vi "Read Logs.vi"() -> ()   [LabVIEW 2020]
panel:
  out "Current Godograph store":cluster{"Y":dbl[], "Y":dbl[]}[](array[cluster])
  out "Voltage Godograph store":cluster{"Y":dbl[], "Y":dbl[]}[](array[cluster])
  out "Current Park Spectrum store":waveform(dbl)[](array[waveform])
  out "Voltage Park Spectrum store":waveform(dbl)[](array[waveform])
  out "Current Spectrum store":waveform(dbl)[](array[waveform])
  out "Voltage Spectrum store":waveform(dbl)[](array[waveform])
  out "Voltage store":waveform(dbl)[](array[waveform])
  out "Current store":waveform(dbl)[](array[waveform])
  in  "Hold":bool
  in  "Plot Selector":u16(ring) items=["Current", "Voltage", "Current Godograph", "Voltage Godograph", "Current Spectrum", "Voltage Spectrum", "Current Park Spectrum", "Voltage Park Spectrum"]
  in  "Choose file":bool
  out "Current Godograph":cluster{"Y":dbl[], "Y":dbl[]}[](graph)
  out "Voltage Godograph":cluster{"Y":dbl[], "Y":dbl[]}[](graph)
  out "Voltage Park Spectrum":waveform(dbl)[](graph)
  out "Current Park Spectrum":waveform(dbl)[](graph)
  out "Current Spectrum":waveform(dbl)[](graph)
  out "Voltage Spectrum":waveform(dbl)[](graph)
  out "Current":waveform(dbl)[](graph)
  out "Voltage":waveform(dbl)[](graph)
  out "error out":errorcluster
types:
  T1 = enum16{"Always On", "Always Off", "Off While Running"}
  T2 = typedef "LVPositionTypeDef.ctl" = cluster{"Left":i32, "Top":i32}
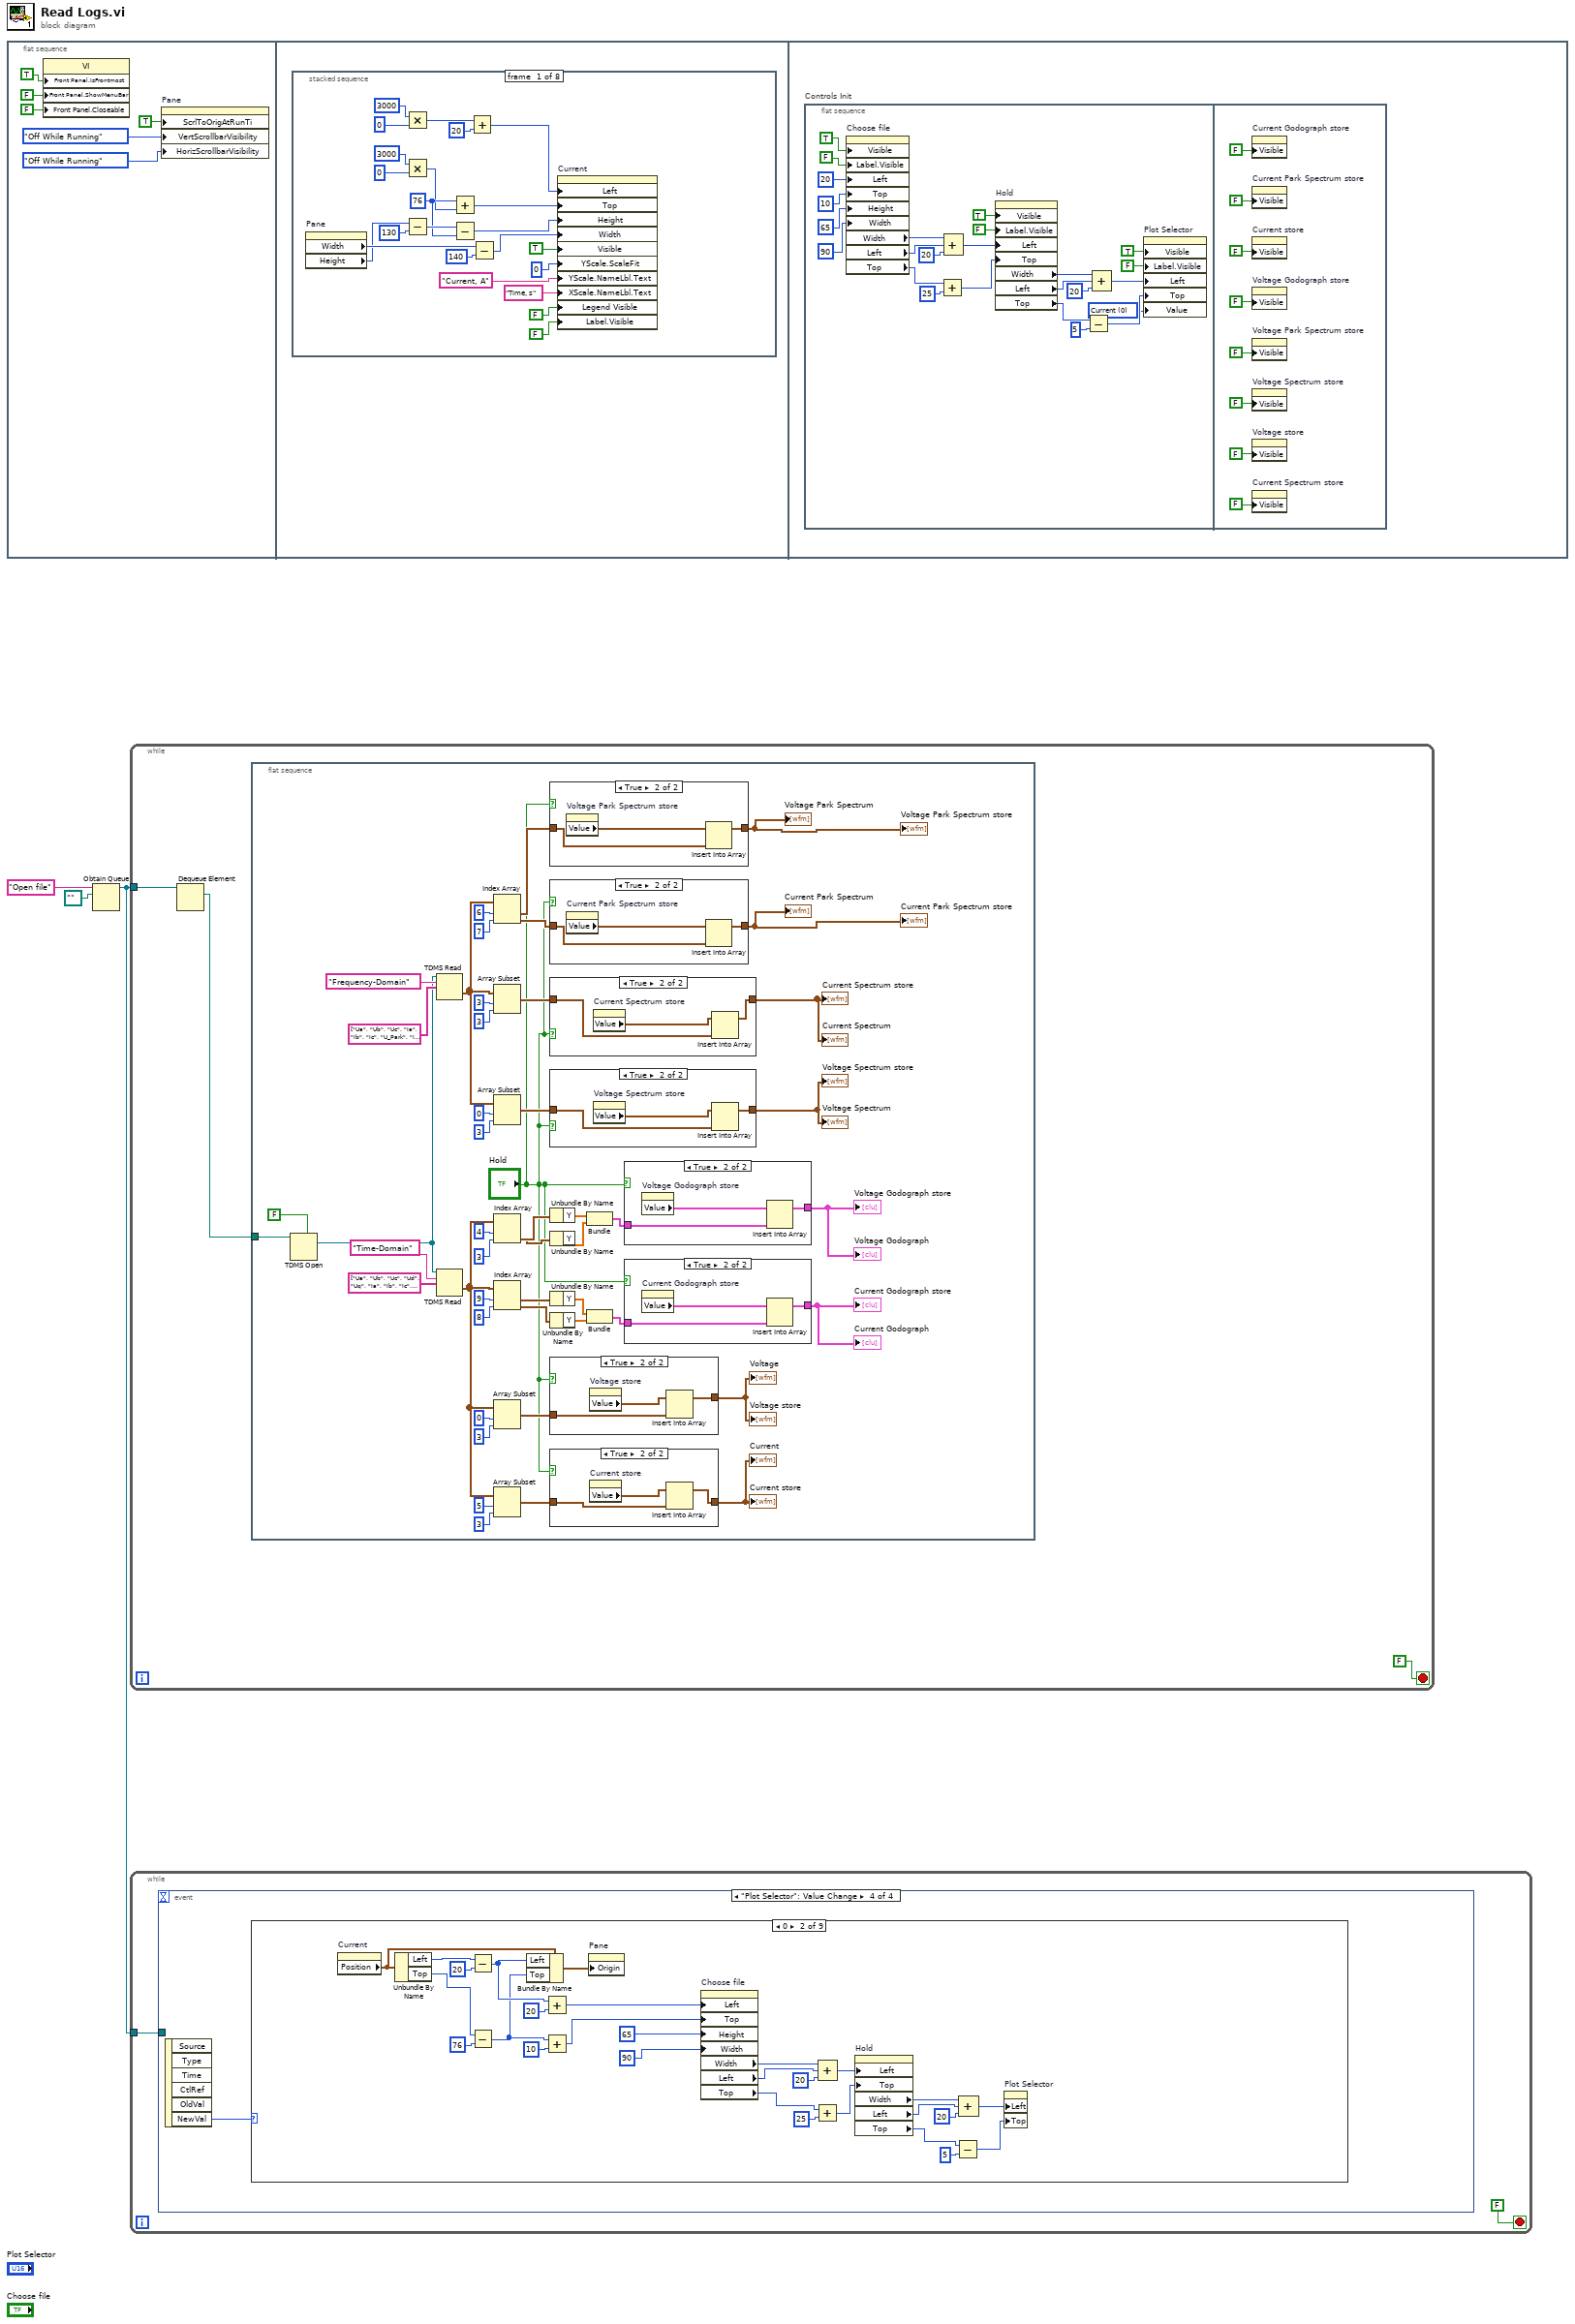
[diagram p0: block diagram]
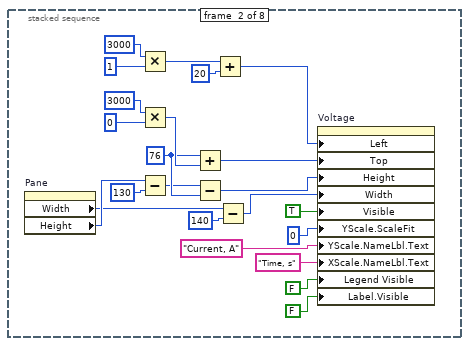
[diagram p2: hidden frame]
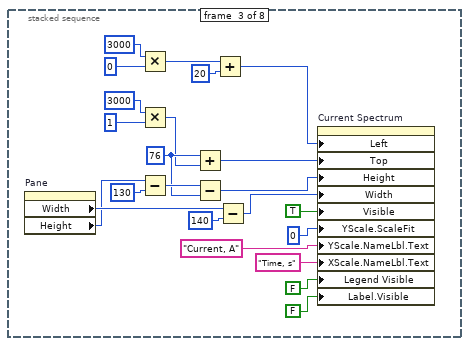
[diagram p3: hidden frame]
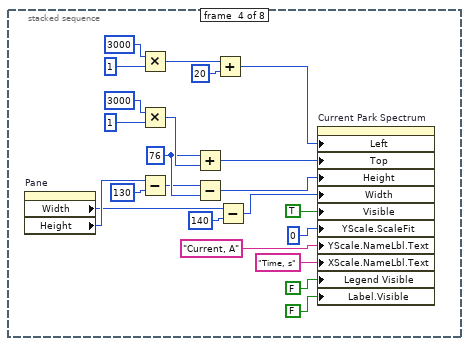
[diagram p4: hidden frame]
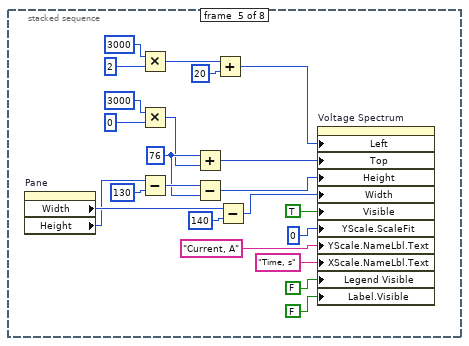
[diagram p5: hidden frame]
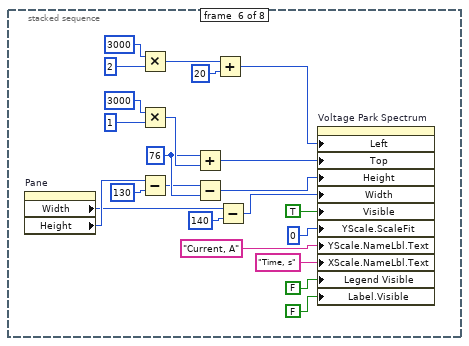
[diagram p6: hidden frame]
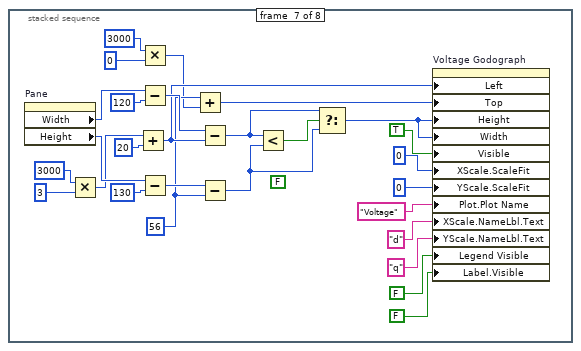
[diagram p7: hidden frame]
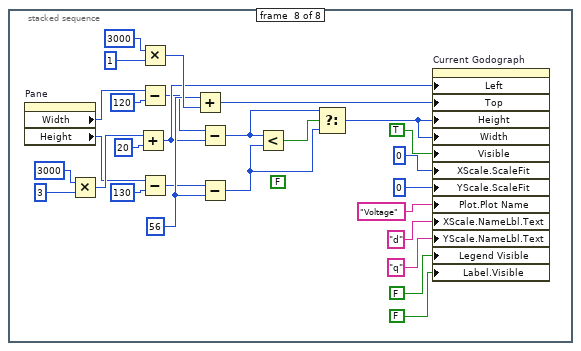
[diagram p8: hidden frame]
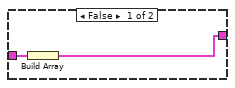
[diagram p9: hidden frame]
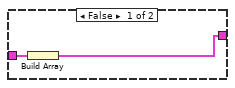
[diagram p10: hidden frame]
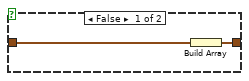
[diagram p11: hidden frame]
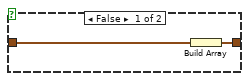
[diagram p12: hidden frame]
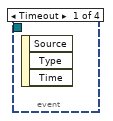
[diagram p17: hidden frame]
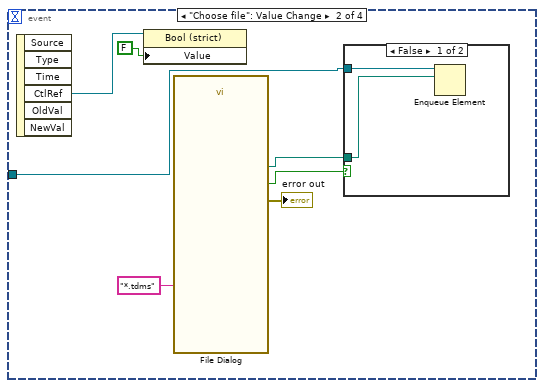
[diagram p18: hidden frame]
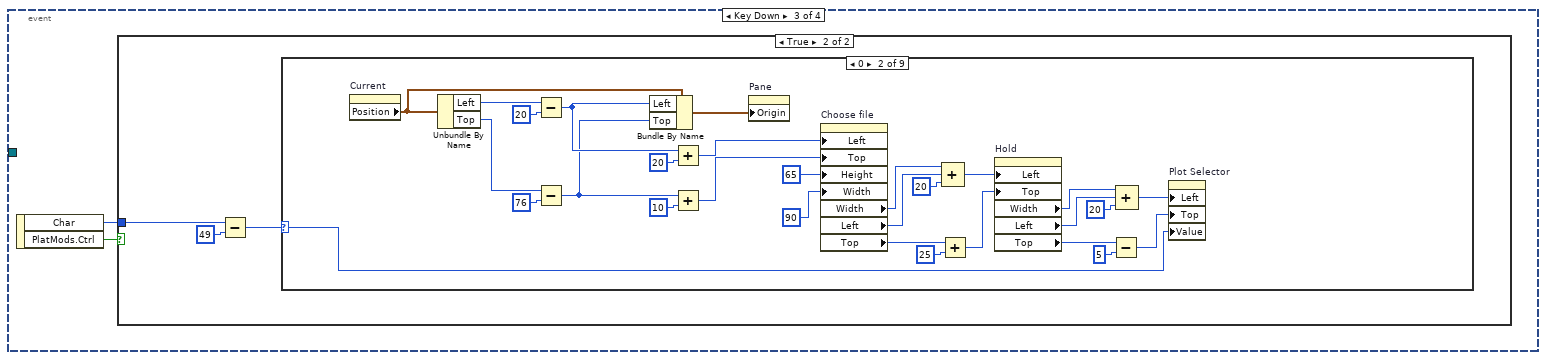
[diagram p20: hidden frame]
diagram:
  n1 = flat-sequence {
    frame #0 {
      n2 = property class="VI"("Front Panel.IsFrontmost"=TRUE ("Front Panel Window:Is Frontmost"), "Front Panel.ShowMenuBar"=FALSE ("Front Panel Window:Show Menu Bar"), "Front Panel.Closeable"=FALSE ("Front Panel Window:Closeable")) -> ()  [unwired: 2 in, 2 out]
      n3 = property on="Pane" class="Pane"("ScrlToOrigAtRunTi"=TRUE ("Scroll To Origin At Run Time"), "VertScrollbarVisibility"=T1."Off While Running" ("Vertical Scrollbar Visibility"), "HorizScrollbarVisibility"=T1."Off While Running" ("Horizontal Scrollbar Visibility")) -> ()  [unwired: 2 in, 2 out]
    }
    frame #1 {
      n4 = stacked-sequence {
        frame #0 {
          w13 = 76 ("Position:Top")
          n5 = property on="Pane" class="Pane"() -> ("Width"=w31:u32, "Height"=w25:u32)  [unwired: 2 in, 2 out]
          n6 = Multiply(x=3000, y=0 ("Position:Left")) -> (x*y=w19:i32)
          n7 = Multiply(x=3000, y=0 ("Position:Left")) -> (x*y=w12:i32)
          n8 = Subtract(x=w25, y=u32 130) -> (x-y=w29:u32)
          n9 = Add(x=w13, y=w12) -> (x+y=w14:i32)
          n10 = Subtract(x=w29, y=w13) -> (x-y=w27:u32)
          n11 = Add(x=w19, y=20 ("Position:Left")) -> (x+y=w21:i32)
          n12 = Subtract(x=w31, y=u32 140) -> (x-y=w11:u32)
          n13 = property on="Current" class="WFGraph (strict)"("Left"=w21, "Top"=w14, "Height"=w27, "Width"=w11, "Visible"=TRUE, "YScale.ScaleFit"=u8 0 ("Y Scale.Scale Fit"), "YScale.NameLbl.Text"="Current, A" ("Y Scale.Name Label.Text"), "XScale.NameLbl.Text"="Time, s" ("X Scale.Name Label.Text"), "Legend Visible"=FALSE ("Legend:Visible"), "Label.Visible"=FALSE) -> ()  [unwired: 2 in, 2 out]
        }
        frame #1 {
          w54 = 76 ("Position:Top")
          n14 = property on="Pane" class="Pane"() -> ("Width"=w36:u32, "Height"=w42:u32)  [unwired: 2 in, 2 out]
          n15 = Multiply(x=3000, y=1 ("Position:Left")) -> (x*y=w48:i32)
          n16 = Multiply(x=3000, y=0 ("Position:Left")) -> (x*y=w55:i32)
          n17 = Subtract(x=w42, y=u32 130) -> (x-y=w38:u32)
          n18 = Add(x=w54, y=w55) -> (x+y=w53:i32)
          n19 = Subtract(x=w38, y=w54) -> (x-y=w40:u32)
          n20 = Add(x=w48, y=20 ("Position:Left")) -> (x+y=w46:i32)
          n21 = Subtract(x=w36, y=u32 140) -> (x-y=w34:u32)
          n22 = property on="Voltage" class="WFGraph (strict)"("Left"=w46, "Top"=w53, "Height"=w40, "Width"=w34, "Visible"=TRUE, "YScale.ScaleFit"=u8 0 ("Y Scale.Scale Fit"), "YScale.NameLbl.Text"="Current, A" ("Y Scale.Name Label.Text"), "XScale.NameLbl.Text"="Time, s" ("X Scale.Name Label.Text"), "Legend Visible"=FALSE ("Legend:Visible"), "Label.Visible"=FALSE) -> ()  [unwired: 2 in, 2 out]
        }
        frame #2 {
          w60 = 76 ("Position:Top")
          n23 = property on="Pane" class="Pane"() -> ("Width"=w77:u32, "Height"=w71:u32)  [unwired: 2 in, 2 out]
          n24 = Multiply(x=3000, y=0 ("Position:Left")) -> (x*y=w65:i32)
          n25 = Multiply(x=3000, y=1 ("Position:Left")) -> (x*y=w59:i32)
          n26 = Subtract(x=w71, y=u32 130) -> (x-y=w75:u32)
          n27 = Add(x=w60, y=w59) -> (x+y=w61:i32)
          n28 = Subtract(x=w75, y=w60) -> (x-y=w73:u32)
          n29 = Add(x=w65, y=20 ("Position:Left")) -> (x+y=w67:i32)
          n30 = Subtract(x=w77, y=u32 140) -> (x-y=w57:u32)
          n31 = property on="Current Spectrum" class="WFGraph (strict)"("Left"=w67, "Top"=w61, "Height"=w73, "Width"=w57, "Visible"=TRUE, "YScale.ScaleFit"=u8 0 ("Y Scale.Scale Fit"), "YScale.NameLbl.Text"="Current, A" ("Y Scale.Name Label.Text"), "XScale.NameLbl.Text"="Time, s" ("X Scale.Name Label.Text"), "Legend Visible"=FALSE ("Legend:Visible"), "Label.Visible"=FALSE) -> ()  [unwired: 2 in, 2 out]
        }
        frame #3 {
          w99 = 76 ("Position:Top")
          n32 = property on="Pane" class="Pane"() -> ("Width"=w82:u32, "Height"=w88:u32)  [unwired: 2 in, 2 out]
          n33 = Multiply(x=3000, y=1 ("Position:Left")) -> (x*y=w94:i32)
          n34 = Multiply(x=3000, y=1 ("Position:Left")) -> (x*y=w100:i32)
          n35 = Subtract(x=w88, y=u32 130) -> (x-y=w84:u32)
          n36 = Add(x=w99, y=w100) -> (x+y=w98:i32)
          n37 = Subtract(x=w84, y=w99) -> (x-y=w86:u32)
          n38 = Add(x=w94, y=20 ("Position:Left")) -> (x+y=w92:i32)
          n39 = Subtract(x=w82, y=u32 140) -> (x-y=w80:u32)
          n40 = property on="Current Park Spectrum" class="WFGraph (strict)"("Left"=w92, "Top"=w98, "Height"=w86, "Width"=w80, "Visible"=TRUE, "YScale.ScaleFit"=u8 0 ("Y Scale.Scale Fit"), "YScale.NameLbl.Text"="Current, A" ("Y Scale.Name Label.Text"), "XScale.NameLbl.Text"="Time, s" ("X Scale.Name Label.Text"), "Legend Visible"=FALSE ("Legend:Visible"), "Label.Visible"=FALSE) -> ()  [unwired: 2 in, 2 out]
        }
        frame #4 {
          w106 = 76 ("Position:Top")
          n41 = property on="Pane" class="Pane"() -> ("Width"=w123:u32, "Height"=w117:u32)  [unwired: 2 in, 2 out]
          n42 = Multiply(x=3000, y=2 ("Position:Left")) -> (x*y=w111:i32)
          n43 = Multiply(x=3000, y=0 ("Position:Left")) -> (x*y=w105:i32)
          n44 = Subtract(x=w117, y=u32 130) -> (x-y=w121:u32)
          n45 = Add(x=w106, y=w105) -> (x+y=w107:i32)
          n46 = Subtract(x=w121, y=w106) -> (x-y=w119:u32)
          n47 = Add(x=w111, y=20 ("Position:Left")) -> (x+y=w113:i32)
          n48 = Subtract(x=w123, y=u32 140) -> (x-y=w103:u32)
          n49 = property on="Voltage Spectrum" class="WFGraph (strict)"("Left"=w113, "Top"=w107, "Height"=w119, "Width"=w103, "Visible"=TRUE, "YScale.ScaleFit"=u8 0 ("Y Scale.Scale Fit"), "YScale.NameLbl.Text"="Current, A" ("Y Scale.Name Label.Text"), "XScale.NameLbl.Text"="Time, s" ("X Scale.Name Label.Text"), "Legend Visible"=FALSE ("Legend:Visible"), "Label.Visible"=FALSE) -> ()  [unwired: 2 in, 2 out]
        }
        frame #5 {
          w145 = 76 ("Position:Top")
          n50 = property on="Pane" class="Pane"() -> ("Width"=w128:u32, "Height"=w134:u32)  [unwired: 2 in, 2 out]
          n51 = Multiply(x=3000, y=2 ("Position:Left")) -> (x*y=w140:i32)
          n52 = Multiply(x=3000, y=1 ("Position:Left")) -> (x*y=w146:i32)
          n53 = Subtract(x=w134, y=u32 130) -> (x-y=w130:u32)
          n54 = Add(x=w145, y=w146) -> (x+y=w144:i32)
          n55 = Subtract(x=w130, y=w145) -> (x-y=w132:u32)
          n56 = Add(x=w140, y=20 ("Position:Left")) -> (x+y=w138:i32)
          n57 = Subtract(x=w128, y=u32 140) -> (x-y=w126:u32)
          n58 = property on="Voltage Park Spectrum" class="WFGraph (strict)"("Left"=w138, "Top"=w144, "Height"=w132, "Width"=w126, "Visible"=TRUE, "YScale.ScaleFit"=u8 0 ("Y Scale.Scale Fit"), "YScale.NameLbl.Text"="Current, A" ("Y Scale.Name Label.Text"), "XScale.NameLbl.Text"="Time, s" ("X Scale.Name Label.Text"), "Legend Visible"=FALSE ("Legend:Visible"), "Label.Visible"=FALSE) -> ()  [unwired: 2 in, 2 out]
        }
        frame #6 {
          (unwired) FALSE ("Visible")
          w150 = 56 ("Position:Top")
          n59 = property on="Pane" class="Pane"() -> ("Width"=w169:u32, "Height"=w166:u32)  [unwired: 2 in, 2 out]
          n60 = Multiply(x=3000, y=3 ("Position:Left")) -> (x*y=w153:i32)
          n61 = Add(x=w153, y=20 ("value")) -> (x+y=w161:i32)
          n62 = Multiply(x=3000, y=0 ("Position:Left")) -> (x*y=w149:i32)
          n63 = Subtract(x=w169, y=u32 120) -> (x-y=w173:u32)
          n64 = Subtract(x=w166, y=u32 130) -> (x-y=w172:u32)
          n65 = Add(x=w150, y=w149) -> (x+y=w148:i32)
          n66 = Subtract(x=w173, y=w161) -> (x-y=w167:u32)
          n67 = Subtract(x=w172, y=w150) -> (x-y=w165:u32)
          n68 = Less?(x=w167, y=w165) -> (x < y?=w170:bool)
          n69 = Select(t=w167, s=w170, f=w165) -> (s? t:f=w168:u32)
          n70 = property on="Voltage Godograph" class="XYGraph (strict)"("Left"=w161, "Top"=w148, "Height"=w168, "Width"=w168, "Visible"=TRUE, "XScale.ScaleFit"=u8 0 ("X Scale.Scale Fit"), "YScale.ScaleFit"=u8 0 ("Y Scale.Scale Fit"), "Plot.Plot Name"="Voltage", "XScale.NameLbl.Text"="d" ("X Scale.Name Label.Text"), "YScale.NameLbl.Text"="q" ("Y Scale.Name Label.Text"), "Legend Visible"=FALSE ("Legend:Visible"), "Label.Visible"=FALSE) -> ()  [unwired: 2 in, 2 out]
        }
        frame #7 {
          (unwired) FALSE ("Visible")
          w201 = 56 ("Position:Top")
          n71 = property on="Pane" class="Pane"() -> ("Width"=w182:u32, "Height"=w185:u32)  [unwired: 2 in, 2 out]
          n72 = Multiply(x=3000, y=3 ("Position:Left")) -> (x*y=w198:i32)
          n73 = Add(x=w198, y=20 ("value")) -> (x+y=w190:i32)
          n74 = Multiply(x=3000, y=1 ("Position:Left")) -> (x*y=w202:i32)
          n75 = Subtract(x=w182, y=u32 120) -> (x-y=w178:u32)
          n76 = Subtract(x=w185, y=u32 130) -> (x-y=w179:u32)
          n77 = Add(x=w201, y=w202) -> (x+y=w203:i32)
          n78 = Subtract(x=w178, y=w190) -> (x-y=w184:u32)
          n79 = Subtract(x=w179, y=w201) -> (x-y=w186:u32)
          n80 = Less?(x=w184, y=w186) -> (x < y?=w181:bool)
          n81 = Select(t=w184, s=w181, f=w186) -> (s? t:f=w183:u32)
          n82 = property on="Current Godograph" class="XYGraph (strict)"("Left"=w190, "Top"=w203, "Height"=w183, "Width"=w183, "Visible"=TRUE, "XScale.ScaleFit"=u8 0 ("X Scale.Scale Fit"), "YScale.ScaleFit"=u8 0 ("Y Scale.Scale Fit"), "Plot.Plot Name"="Voltage", "XScale.NameLbl.Text"="d" ("X Scale.Name Label.Text"), "YScale.NameLbl.Text"="q" ("Y Scale.Name Label.Text"), "Legend Visible"=FALSE ("Legend:Visible"), "Label.Visible"=FALSE) -> ()  [unwired: 2 in, 2 out]
        }
      }
    }
    frame #2 {
      n83 = flat-sequence "Controls Init" {
        frame #0 {
          w204 = u16 0 items=["Current", "Voltage", "Current Godograph", "Voltage Godograph", "Current Spectrum", "Voltage Spectrum", "Current Park Spectrum", "Voltage Park Spectrum"] ("Plot Selector")
          n84 = property on="Choose file" class="Bool (strict)"("Visible"=TRUE, "Label.Visible"=FALSE, "Left"=20 ("Position:Left"), "Top"=10 ("Position:Top"), "Height"=u32 65 ("Button Size:Height"), "Width"=u32 90 ("Button Size:Width")) -> ("Width"=w215:u32, "Left"=w214:i32, "Top"=w210:i32)  [unwired: 2 in, 2 out]
          n85 = Add(x=w210, y=25) -> (x+y=w208:i32)
          n86 = Compound Arithmetic op=ADD(w215, w214, 20 ("value")) -> (w213:u32)
          n87 = property on="Hold" class="Bool (strict)"("Visible"=TRUE, "Label.Visible"=FALSE, "Left"=w213, "Top"=w208) -> ("Width"=w212:u32, "Left"=w211:i32, "Top"=w207:i32)  [unwired: 2 in, 2 out]
          n88 = Subtract(x=w207, y=5) -> (x-y=w205:i32)
          n89 = Compound Arithmetic op=ADD(w212, w211, 20 ("value")) -> (w221:u32)
          n90 = property on="Plot Selector" class="Ring (strict)"("Visible"=TRUE, "Label.Visible"=FALSE, "Left"=w221, "Top"=w205, "Value"=w204) -> ()  [unwired: 2 in, 2 out]
        }
        frame #1 {
          n91 = property on="Current Godograph store" class="Arr (strict)"("Visible"=FALSE) -> ()  [unwired: 2 in, 2 out]
          n92 = property on="Current Park Spectrum store" class="Arr (strict)"("Visible"=FALSE) -> ()  [unwired: 2 in, 2 out]
          n93 = property on="Current store" class="Arr (strict)"("Visible"=FALSE) -> ()  [unwired: 2 in, 2 out]
          n94 = property on="Voltage Godograph store" class="Arr (strict)"("Visible"=FALSE) -> ()  [unwired: 2 in, 2 out]
          n95 = property on="Voltage Park Spectrum store" class="Arr (strict)"("Visible"=FALSE) -> ()  [unwired: 2 in, 2 out]
          n96 = property on="Voltage Spectrum store" class="Arr (strict)"("Visible"=FALSE) -> ()  [unwired: 2 in, 2 out]
          n97 = property on="Voltage store" class="Arr (strict)"("Visible"=FALSE) -> ()  [unwired: 2 in, 2 out]
          n98 = property on="Current Spectrum store" class="Arr (strict)"("Visible"=FALSE) -> ()  [unwired: 2 in, 2 out]
        }
      }
    }
  }
  n99 = Obtain Queue(name (unnamed)="Open file", element data type=path "") -> (queue out=w1:refnum<queue>)  [unwired: 3 in, 2 out]
  n100 = while {
    tunnel: w1 -> [w239]
    stop <- FALSE stop-if-true
    n101 = Dequeue Element(queue=w239) -> (element=w237:path)  [unwired: 2 in, 3 out]
    n102 = flat-sequence {
      tunnel: w237 -> [w260]
      frame #0 {
        n103 = TDMS Open(5:FALSE ("create index file? (T)"), 11:w260) -> (3:w257:refnum<k34>)  [unwired: 5 in, 1 out]
        n104 = TDMS Read(0:w257, 5:"Frequency-Domain" ("group name in"), 7:string[] ["Ua", "Ub", "Uc", "Ia", "Ib", "Ic", "U_Park", "I_Park"] ("channel name(s) in")) -> (10:w265:waveform(dbl)[])  [unwired: 5 in, 5 out]
        n105 = TDMS Read(0:w257, 5:"Time-Domain" ("group name in"), 7:string[] ["Ua", "Ub", "Uc", "Ud", "Uq", "Ia", "Ib", "Ic", "Id", "Iq"] ("channel name(s) in")) -> (10:w269:waveform(dbl)[])  [unwired: 5 in, 5 out]
        n106 = Index Array(array=w265, index #1=6 ("index"), index #2=7 ("index")) -> (element #1=w248:waveform(dbl), element #2=w246:waveform(dbl))
        n107 = Array Subset(array=w265, index=3, length=3) -> (w250:waveform(dbl)[])
        n108 = Array Subset(array=w265, index=0, length=3) -> (w252:waveform(dbl)[])
        n109 = Index Array(array=w269, index #1=4 ("index"), index #2=3 ("index")) -> (element #1=w279:waveform(dbl), element #2=w277:waveform(dbl))
        n110 = Index Array(array=w269, index #1=9 ("index"), index #2=8 ("index")) -> (element #1=w272:waveform(dbl), element #2=w274:waveform(dbl))
        n111 = Array Subset(array=w269, index=0, length=3) -> (w254:waveform(dbl)[])
        n112 = Array Subset(array=w269, index=5, length=3) -> (w256:waveform(dbl)[])
        n113 = case shown="True" "Hold" {
          tunnel: [w304 w306] -> w247
          tunnel: w248 -> [w303 w305]
          frame False {
            n114 = Build Array(w303) -> (w304:waveform(dbl)[])
          }
          frame True {
            n115 = property on="Voltage Park Spectrum store" class="Arr (strict)"() -> ("Value"=w307:waveform(dbl)[])  [unwired: 2 in, 2 out]
            n116 = Insert Into Array(array=w307, new element=w305) -> (w306:waveform(dbl)[])  [unwired: 1 in]
          }
        }
        "Voltage Park Spectrum" <- w247
        "Voltage Park Spectrum store" <- w247
        n117 = case shown="True" "Hold" {
          tunnel: [w299 w301] -> w245
          tunnel: w246 -> [w298 w300]
          frame False {
            n118 = Build Array(w298) -> (w299:waveform(dbl)[])
          }
          frame True {
            n119 = property on="Current Park Spectrum store" class="Arr (strict)"() -> ("Value"=w302:waveform(dbl)[])  [unwired: 2 in, 2 out]
            n120 = Insert Into Array(array=w302, new element=w300) -> (w301:waveform(dbl)[])  [unwired: 1 in]
          }
        }
        "Current Park Spectrum" <- w245
        "Current Park Spectrum store" <- w245
        n121 = case shown="True" "Hold" {
          tunnel: [w308 w310] -> w249
          tunnel: w250 -> [w308 w309]
          frame False {
          }
          frame True {
            n122 = property on="Current Spectrum store" class="Arr (strict)"() -> ("Value"=w311:waveform(dbl)[])  [unwired: 2 in, 2 out]
            n123 = Insert Into Array(array=w311, new element=w309) -> (w310:waveform(dbl)[])  [unwired: 1 in]
          }
        }
        "Current Spectrum" <- w249
        "Current Spectrum store" <- w249
        n124 = case shown="True" "Hold" {
          tunnel: [w312 w314] -> w251
          tunnel: w252 -> [w312 w313]
          frame False {
          }
          frame True {
            n125 = property on="Voltage Spectrum store" class="Arr (strict)"() -> ("Value"=w315:waveform(dbl)[])  [unwired: 2 in, 2 out]
            n126 = Insert Into Array(array=w315, new element=w313) -> (w314:waveform(dbl)[])  [unwired: 1 in]
          }
        }
        "Voltage Spectrum" <- w251
        "Voltage Spectrum store" <- w251
        n127 = Unbundle By Name(w279) -> ("Y"=w278:dbl[])
        n128 = Unbundle By Name(w277) -> ("Y"=w276:dbl[])
        n129 = Unbundle By Name(w272) -> ("Y"=w273:dbl[])
        n130 = Unbundle By Name(w274) -> ("Y"=w275:dbl[])
        n131 = case shown="True" "Hold" {
          tunnel: w254 -> [w316 w319]
          tunnel: [w316 w317] -> w253
          frame False {
          }
          frame True {
            n132 = property on="Voltage store" class="Arr (strict)"() -> ("Value"=w318:waveform(dbl)[])  [unwired: 2 in, 2 out]
            n133 = Insert Into Array(array=w318, new element=w319) -> (w317:waveform(dbl)[])  [unwired: 1 in]
          }
        }
        "Voltage" <- w253
        "Voltage store" <- w253
        n134 = case shown="True" "Hold" {
          tunnel: w256 -> [w320 w323]
          tunnel: [w320 w321] -> w255
          frame False {
          }
          frame True {
            n135 = property on="Current store" class="Arr (strict)"() -> ("Value"=w322:waveform(dbl)[])  [unwired: 2 in, 2 out]
            n136 = Insert Into Array(array=w322, new element=w323) -> (w321:waveform(dbl)[])  [unwired: 1 in]
          }
        }
        "Current" <- w255
        "Current store" <- w255
        n137 = Bundle("Y"=w278, "Y"=w276) -> (w244:cluster{"Y":dbl[], "Y":dbl[]})  [unwired: 1 in]
        n138 = Bundle("Y"=w273, "Y"=w275) -> (w241:cluster{"Y":dbl[], "Y":dbl[]})  [unwired: 1 in]
        n139 = case shown="True" "Hold" {
          tunnel: w244 -> [w294 w297]
          tunnel: [w293 w295] -> w243
          frame False {
            n140 = Build Array(w294) -> (w293:cluster{"Y":dbl[], "Y":dbl[]}[])
          }
          frame True {
            n141 = property on="Voltage Godograph store" class="Arr (strict)"() -> ("Value"=w296:cluster{"Y":dbl[], "Y":dbl[]}[])  [unwired: 2 in, 2 out]
            n142 = Insert Into Array(array=w296, new element=w297) -> (w295:cluster{"Y":dbl[], "Y":dbl[]}[])  [unwired: 1 in]
          }
        }
        "Voltage Godograph" <- w243
        "Voltage Godograph store" <- w243
        n143 = case shown="True" "Hold" {
          tunnel: w241 -> [w289 w292]
          tunnel: [w288 w290] -> w242
          frame False {
            n144 = Build Array(w289) -> (w288:cluster{"Y":dbl[], "Y":dbl[]}[])
          }
          frame True {
            n145 = property on="Current Godograph store" class="Arr (strict)"() -> ("Value"=w291:cluster{"Y":dbl[], "Y":dbl[]}[])  [unwired: 2 in, 2 out]
            n146 = Insert Into Array(array=w291, new element=w292) -> (w290:cluster{"Y":dbl[], "Y":dbl[]}[])  [unwired: 1 in]
          }
        }
        "Current Godograph" <- w242
        "Current Godograph store" <- w242
      }
    }
  }
  n147 = while {
    tunnel: w1 -> [w324]
    stop <- FALSE stop-if-true
    n148 = event shown="[3] \"Plot Selector\": Value Change" {
      selector: _ -> [_ _ _ _]
      dyn-events: _ -> [_ _ _ _]
      timeout: _ -> [_ _ _ _]
      tunnel: w324 -> [_ w327 _ _]
      event Timeout {
        n149 = event-data() -> ()  [unwired: 1 in, 3 out]
      }
      event "Choose file": Value Change {
        n150 = event-data() -> ("CtlRef"=w326:refnum<vi>)  [unwired: 1 in, 5 out]
        n151 = property on="Property Node" class="Bool (strict)"(reference=w326, "Value"=FALSE ("Choose file")) -> ()  [unwired: 1 in, 2 out]
        n152 = call "File Dialog"("pattern (all files)"="*.tdms") -> ("selected path"=w328:path, "cancelled"=w329:bool, "error out"=→"error out":errorcluster)  [unwired: 11 in, 1 out]
        n153 = case shown="False" w329 {
          tunnel: w328 -> [w333 _]
          tunnel: w327 -> [w334 _]
          frame False {
            n154 = Enqueue Element(queue=w334, element=w333) -> ()  [unwired: 2 in, 3 out]
          }
          frame True {
          }
        }
      }
      event Key Down {
        n155 = event-data() -> ("Char"=w336:i16, "PlatMods.Ctrl"=w335:bool)  [unwired: 1 in]
        n156 = case shown="True" w335 {
          tunnel: w336 -> [_ w339]
          frame False {
          }
          frame True {
            n157 = Subtract(x=w339, y=i16 49) -> (x-y=w337:i16)
            n158 = case shown="0" w337 {
              selector: w337 -> [_ w340 w369 w398 w427 w456 w485 w514 w543]
              frame Default {
              }
              frame 0 {
                n159 = property on="Current" class="WFGraph (strict)"() -> ("Position"=w365:T2)  [unwired: 2 in, 2 out]
                n160 = Unbundle By Name(w365) -> ("Left"=w364:i32, "Top"=w363:i32)
                n161 = Subtract(x=w364, y=20) -> (x-y=w342:i32)
                n162 = Subtract(x=w363, y=76) -> (x-y=w341:i32)
                n163 = Bundle By Name(cluster=w365, "Left"=w342, "Top"=w341) -> (w366:T2)
                n164 = Add(x=w342, y=20 ("Position:Left")) -> (x+y=w344:i32)
                n165 = Add(x=w341, y=10 ("Position:Top")) -> (x+y=w343:i32)
                n166 = property on="Pane" class="Pane"("Origin"=w366) -> ()  [unwired: 2 in, 2 out]
                n167 = property on="Choose file" class="Bool (strict)"("Left"=w344, "Top"=w343, "Height"=u32 65 ("Button Size:Height"), "Width"=u32 90 ("Button Size:Width")) -> ("Width"=w357:u32, "Left"=w356:i32, "Top"=w352:i32)  [unwired: 2 in, 2 out]
                n168 = Add(x=w352, y=25) -> (x+y=w350:i32)
                n169 = Compound Arithmetic op=ADD(w357, w356, 20 ("value")) -> (w355:u32)
                n170 = property on="Hold" class="Bool (strict)"("Left"=w355, "Top"=w350) -> ("Width"=w354:u32, "Left"=w353:i32, "Top"=w349:i32)  [unwired: 2 in, 2 out]
                n171 = Subtract(x=w349, y=5) -> (x-y=w347:i32)
                n172 = Compound Arithmetic op=ADD(w354, w353, 20 ("value")) -> (w361:u32)
                n173 = property on="Plot Selector" class="Ring (strict)"("Left"=w361, "Top"=w347, "Value"=w340) -> ()  [unwired: 2 in, 2 out]
              }
              frame 1 {
                n174 = property on="Voltage" class="WFGraph (strict)"() -> ("Position"=w394:T2)  [unwired: 2 in, 2 out]
                n175 = Unbundle By Name(w394) -> ("Left"=w393:i32, "Top"=w392:i32)
                n176 = Subtract(x=w393, y=20) -> (x-y=w371:i32)
                n177 = Subtract(x=w392, y=76) -> (x-y=w370:i32)
                n178 = Bundle By Name(cluster=w394, "Left"=w371, "Top"=w370) -> (w395:T2)
                n179 = Add(x=w371, y=20 ("Position:Left")) -> (x+y=w373:i32)
                n180 = Add(x=w370, y=10 ("Position:Top")) -> (x+y=w372:i32)
                n181 = property on="Pane" class="Pane"("Origin"=w395) -> ()  [unwired: 2 in, 2 out]
                n182 = property on="Choose file" class="Bool (strict)"("Left"=w373, "Top"=w372, "Height"=u32 65 ("Button Size:Height"), "Width"=u32 90 ("Button Size:Width")) -> ("Width"=w386:u32, "Left"=w385:i32, "Top"=w381:i32)  [unwired: 2 in, 2 out]
                n183 = Add(x=w381, y=25) -> (x+y=w379:i32)
                n184 = Compound Arithmetic op=ADD(w386, w385, 20 ("value")) -> (w384:u32)
                n185 = property on="Hold" class="Bool (strict)"("Left"=w384, "Top"=w379) -> ("Width"=w383:u32, "Left"=w382:i32, "Top"=w378:i32)  [unwired: 2 in, 2 out]
                n186 = Subtract(x=w378, y=5) -> (x-y=w376:i32)
                n187 = Compound Arithmetic op=ADD(w383, w382, 20 ("value")) -> (w390:u32)
                n188 = property on="Plot Selector" class="Ring (strict)"("Left"=w390, "Top"=w376, "Value"=w369) -> ()  [unwired: 2 in, 2 out]
              }
              frame 2 {
                n189 = property on="Current Godograph" class="XYGraph (strict)"() -> ("Position"=w423:T2)  [unwired: 2 in, 2 out]
                n190 = Unbundle By Name(w423) -> ("Left"=w422:i32, "Top"=w421:i32)
                n191 = Subtract(x=w422, y=20) -> (x-y=w400:i32)
                n192 = Subtract(x=w421, y=76) -> (x-y=w399:i32)
                n193 = Bundle By Name(cluster=w423, "Left"=w400, "Top"=w399) -> (w424:T2)
                n194 = Add(x=w400, y=20 ("Position:Left")) -> (x+y=w402:i32)
                n195 = Add(x=w399, y=10 ("Position:Top")) -> (x+y=w401:i32)
                n196 = property on="Pane" class="Pane"("Origin"=w424) -> ()  [unwired: 2 in, 2 out]
                n197 = property on="Choose file" class="Bool (strict)"("Left"=w402, "Top"=w401, "Height"=u32 65 ("Button Size:Height"), "Width"=u32 90 ("Button Size:Width")) -> ("Width"=w415:u32, "Left"=w414:i32, "Top"=w410:i32)  [unwired: 2 in, 2 out]
                n198 = Add(x=w410, y=25) -> (x+y=w408:i32)
                n199 = Compound Arithmetic op=ADD(w415, w414, 20 ("value")) -> (w413:u32)
                n200 = property on="Hold" class="Bool (strict)"("Left"=w413, "Top"=w408) -> ("Width"=w412:u32, "Left"=w411:i32, "Top"=w407:i32)  [unwired: 2 in, 2 out]
                n201 = Subtract(x=w407, y=5) -> (x-y=w405:i32)
                n202 = Compound Arithmetic op=ADD(w412, w411, 20 ("value")) -> (w419:u32)
                n203 = property on="Plot Selector" class="Ring (strict)"("Left"=w419, "Top"=w405, "Value"=w398) -> ()  [unwired: 2 in, 2 out]
              }
              frame 3 {
                n204 = property on="Voltage Godograph" class="XYGraph (strict)"() -> ("Position"=w454:T2)  [unwired: 2 in, 2 out]
                n205 = Unbundle By Name(w454) -> ("Left"=w453:i32, "Top"=w452:i32)
                n206 = Subtract(x=w453, y=20) -> (x-y=w429:i32)
                n207 = Subtract(x=w452, y=76) -> (x-y=w428:i32)
                n208 = Bundle By Name(cluster=w454, "Left"=w429, "Top"=w428) -> (w455:T2)
                n209 = Add(x=w429, y=20 ("Position:Left")) -> (x+y=w431:i32)
                n210 = Add(x=w428, y=10 ("Position:Top")) -> (x+y=w430:i32)
                n211 = property on="Pane" class="Pane"("Origin"=w455) -> ()  [unwired: 2 in, 2 out]
                n212 = property on="Choose file" class="Bool (strict)"("Left"=w431, "Top"=w430, "Height"=u32 65 ("Button Size:Height"), "Width"=u32 90 ("Button Size:Width")) -> ("Width"=w444:u32, "Left"=w443:i32, "Top"=w439:i32)  [unwired: 2 in, 2 out]
                n213 = Add(x=w439, y=25) -> (x+y=w437:i32)
                n214 = Compound Arithmetic op=ADD(w444, w443, 20 ("value")) -> (w442:u32)
                n215 = property on="Hold" class="Bool (strict)"("Left"=w442, "Top"=w437) -> ("Width"=w441:u32, "Left"=w440:i32, "Top"=w436:i32)  [unwired: 2 in, 2 out]
                n216 = Subtract(x=w436, y=5) -> (x-y=w434:i32)
                n217 = Compound Arithmetic op=ADD(w441, w440, 20 ("value")) -> (w448:u32)
                n218 = property on="Plot Selector" class="Ring (strict)"("Left"=w448, "Top"=w434, "Value"=w427) -> ()  [unwired: 2 in, 2 out]
              }
              frame 4 {
                n219 = property on="Current Spectrum" class="WFGraph (strict)"() -> ("Position"=w481:T2)  [unwired: 2 in, 2 out]
                n220 = Unbundle By Name(w481) -> ("Left"=w480:i32, "Top"=w479:i32)
                n221 = Subtract(x=w480, y=20) -> (x-y=w458:i32)
                n222 = Subtract(x=w479, y=76) -> (x-y=w457:i32)
                n223 = Bundle By Name(cluster=w481, "Left"=w458, "Top"=w457) -> (w482:T2)
                n224 = Add(x=w458, y=20 ("Position:Left")) -> (x+y=w460:i32)
                n225 = Add(x=w457, y=10 ("Position:Top")) -> (x+y=w459:i32)
                n226 = property on="Pane" class="Pane"("Origin"=w482) -> ()  [unwired: 2 in, 2 out]
                n227 = property on="Choose file" class="Bool (strict)"("Left"=w460, "Top"=w459, "Height"=u32 65 ("Button Size:Height"), "Width"=u32 90 ("Button Size:Width")) -> ("Width"=w473:u32, "Left"=w472:i32, "Top"=w468:i32)  [unwired: 2 in, 2 out]
                n228 = Add(x=w468, y=25) -> (x+y=w466:i32)
                n229 = Compound Arithmetic op=ADD(w473, w472, 20 ("value")) -> (w471:u32)
                n230 = property on="Hold" class="Bool (strict)"("Left"=w471, "Top"=w466) -> ("Width"=w470:u32, "Left"=w469:i32, "Top"=w465:i32)  [unwired: 2 in, 2 out]
                n231 = Subtract(x=w465, y=5) -> (x-y=w463:i32)
                n232 = Compound Arithmetic op=ADD(w470, w469, 20 ("value")) -> (w477:u32)
                n233 = property on="Plot Selector" class="Ring (strict)"("Left"=w477, "Top"=w463, "Value"=w456) -> ()  [unwired: 2 in, 2 out]
              }
              frame 5 {
                n234 = property on="Voltage Spectrum" class="WFGraph (strict)"() -> ("Position"=w510:T2)  [unwired: 2 in, 2 out]
                n235 = Unbundle By Name(w510) -> ("Left"=w509:i32, "Top"=w508:i32)
                n236 = Subtract(x=w509, y=20) -> (x-y=w487:i32)
                n237 = Subtract(x=w508, y=76) -> (x-y=w486:i32)
                n238 = Bundle By Name(cluster=w510, "Left"=w487, "Top"=w486) -> (w511:T2)
                n239 = Add(x=w487, y=20 ("Position:Left")) -> (x+y=w489:i32)
                n240 = Add(x=w486, y=10 ("Position:Top")) -> (x+y=w488:i32)
                n241 = property on="Pane" class="Pane"("Origin"=w511) -> ()  [unwired: 2 in, 2 out]
                n242 = property on="Choose file" class="Bool (strict)"("Left"=w489, "Top"=w488, "Height"=u32 65 ("Button Size:Height"), "Width"=u32 90 ("Button Size:Width")) -> ("Width"=w502:u32, "Left"=w501:i32, "Top"=w497:i32)  [unwired: 2 in, 2 out]
                n243 = Add(x=w497, y=25) -> (x+y=w495:i32)
                n244 = Compound Arithmetic op=ADD(w502, w501, 20 ("value")) -> (w500:u32)
                n245 = property on="Hold" class="Bool (strict)"("Left"=w500, "Top"=w495) -> ("Width"=w499:u32, "Left"=w498:i32, "Top"=w494:i32)  [unwired: 2 in, 2 out]
                n246 = Subtract(x=w494, y=5) -> (x-y=w492:i32)
                n247 = Compound Arithmetic op=ADD(w499, w498, 20 ("value")) -> (w506:u32)
                n248 = property on="Plot Selector" class="Ring (strict)"("Left"=w506, "Top"=w492, "Value"=w485) -> ()  [unwired: 2 in, 2 out]
              }
              frame 6 {
                n249 = property on="Current Park Spectrum" class="WFGraph (strict)"() -> ("Position"=w539:T2)  [unwired: 2 in, 2 out]
                n250 = Unbundle By Name(w539) -> ("Left"=w538:i32, "Top"=w537:i32)
                n251 = Subtract(x=w538, y=20) -> (x-y=w516:i32)
                n252 = Subtract(x=w537, y=76) -> (x-y=w515:i32)
                n253 = Bundle By Name(cluster=w539, "Left"=w516, "Top"=w515) -> (w540:T2)
                n254 = Add(x=w516, y=20 ("Position:Left")) -> (x+y=w518:i32)
                n255 = Add(x=w515, y=10 ("Position:Top")) -> (x+y=w517:i32)
                n256 = property on="Pane" class="Pane"("Origin"=w540) -> ()  [unwired: 2 in, 2 out]
                n257 = property on="Choose file" class="Bool (strict)"("Left"=w518, "Top"=w517, "Height"=u32 65 ("Button Size:Height"), "Width"=u32 90 ("Button Size:Width")) -> ("Width"=w531:u32, "Left"=w530:i32, "Top"=w526:i32)  [unwired: 2 in, 2 out]
                n258 = Add(x=w526, y=25) -> (x+y=w524:i32)
                n259 = Compound Arithmetic op=ADD(w531, w530, 20 ("value")) -> (w529:u32)
                n260 = property on="Hold" class="Bool (strict)"("Left"=w529, "Top"=w524) -> ("Width"=w528:u32, "Left"=w527:i32, "Top"=w523:i32)  [unwired: 2 in, 2 out]
                n261 = Subtract(x=w523, y=5) -> (x-y=w521:i32)
                n262 = Compound Arithmetic op=ADD(w528, w527, 20 ("value")) -> (w535:u32)
                n263 = property on="Plot Selector" class="Ring (strict)"("Left"=w535, "Top"=w521, "Value"=w514) -> ()  [unwired: 2 in, 2 out]
              }
              frame 7 {
                n264 = property on="Voltage Park Spectrum" class="WFGraph (strict)"() -> ("Position"=w568:T2)  [unwired: 2 in, 2 out]
                n265 = Unbundle By Name(w568) -> ("Left"=w567:i32, "Top"=w566:i32)
                n266 = Subtract(x=w567, y=20) -> (x-y=w547:i32)
                n267 = Subtract(x=w566, y=76) -> (x-y=w546:i32)
                n268 = Bundle By Name(cluster=w568, "Left"=w547, "Top"=w546) -> (w569:T2)
                n269 = Add(x=w547, y=20 ("Position:Left")) -> (x+y=w545:i32)
                n270 = Add(x=w546, y=10 ("Position:Top")) -> (x+y=w544:i32)
                n271 = property on="Pane" class="Pane"("Origin"=w569) -> ()  [unwired: 2 in, 2 out]
                n272 = property on="Choose file" class="Bool (strict)"("Left"=w545, "Top"=w544, "Height"=u32 65 ("Button Size:Height"), "Width"=u32 90 ("Button Size:Width")) -> ("Width"=w560:u32, "Left"=w559:i32, "Top"=w555:i32)  [unwired: 2 in, 2 out]
                n273 = Add(x=w555, y=25) -> (x+y=w553:i32)
                n274 = Compound Arithmetic op=ADD(w560, w559, 20 ("value")) -> (w558:u32)
                n275 = property on="Hold" class="Bool (strict)"("Left"=w558, "Top"=w553) -> ("Width"=w557:u32, "Left"=w556:i32, "Top"=w552:i32)  [unwired: 2 in, 2 out]
                n276 = Subtract(x=w552, y=5) -> (x-y=w550:i32)
                n277 = Compound Arithmetic op=ADD(w557, w556, 20 ("value")) -> (w564:u32)
                n278 = property on="Plot Selector" class="Ring (strict)"("Left"=w564, "Top"=w550, "Value"=w543) -> ()  [unwired: 2 in, 2 out]
              }
            }
          }
        }
      }
      event "Plot Selector": Value Change {
        n279 = event-data() -> ("NewVal"=w572:u16)  [unwired: 1 in, 5 out]
        n280 = case shown="0" w572 {
          frame Default {
          }
          frame 0 {
            n281 = property on="Current" class="WFGraph (strict)"() -> ("Position"=w597:T2)  [unwired: 2 in, 2 out]
            n282 = Unbundle By Name(w597) -> ("Left"=w596:i32, "Top"=w595:i32)
            n283 = Subtract(x=w596, y=20) -> (x-y=w574:i32)
            n284 = Subtract(x=w595, y=76) -> (x-y=w573:i32)
            n285 = Bundle By Name(cluster=w597, "Left"=w574, "Top"=w573) -> (w598:T2)
            n286 = Add(x=w574, y=20 ("Position:Left")) -> (x+y=w576:i32)
            n287 = Add(x=w573, y=10 ("Position:Top")) -> (x+y=w575:i32)
            n288 = property on="Pane" class="Pane"("Origin"=w598) -> ()  [unwired: 2 in, 2 out]
            n289 = property on="Choose file" class="Bool (strict)"("Left"=w576, "Top"=w575, "Height"=u32 65 ("Button Size:Height"), "Width"=u32 90 ("Button Size:Width")) -> ("Width"=w589:u32, "Left"=w588:i32, "Top"=w584:i32)  [unwired: 2 in, 2 out]
            n290 = Add(x=w584, y=25) -> (x+y=w582:i32)
            n291 = Compound Arithmetic op=ADD(w589, w588, 20 ("value")) -> (w587:u32)
            n292 = property on="Hold" class="Bool (strict)"("Left"=w587, "Top"=w582) -> ("Width"=w586:u32, "Left"=w585:i32, "Top"=w581:i32)  [unwired: 2 in, 2 out]
            n293 = Subtract(x=w581, y=5) -> (x-y=w579:i32)
            n294 = Compound Arithmetic op=ADD(w586, w585, 20 ("value")) -> (w593:u32)
            n295 = property on="Plot Selector" class="Ring (strict)"("Left"=w593, "Top"=w579) -> ()  [unwired: 2 in, 2 out]
          }
          frame 1 {
            n296 = property on="Voltage" class="WFGraph (strict)"() -> ("Position"=w625:T2)  [unwired: 2 in, 2 out]
            n297 = Unbundle By Name(w625) -> ("Left"=w624:i32, "Top"=w623:i32)
            n298 = Subtract(x=w624, y=20) -> (x-y=w602:i32)
            n299 = Subtract(x=w623, y=76) -> (x-y=w601:i32)
            n300 = Bundle By Name(cluster=w625, "Left"=w602, "Top"=w601) -> (w626:T2)
            n301 = Add(x=w602, y=20 ("Position:Left")) -> (x+y=w604:i32)
            n302 = Add(x=w601, y=10 ("Position:Top")) -> (x+y=w603:i32)
            n303 = property on="Pane" class="Pane"("Origin"=w626) -> ()  [unwired: 2 in, 2 out]
            n304 = property on="Choose file" class="Bool (strict)"("Left"=w604, "Top"=w603, "Height"=u32 65 ("Button Size:Height"), "Width"=u32 90 ("Button Size:Width")) -> ("Width"=w617:u32, "Left"=w616:i32, "Top"=w612:i32)  [unwired: 2 in, 2 out]
            n305 = Add(x=w612, y=25) -> (x+y=w610:i32)
            n306 = Compound Arithmetic op=ADD(w617, w616, 20 ("value")) -> (w615:u32)
            n307 = property on="Hold" class="Bool (strict)"("Left"=w615, "Top"=w610) -> ("Width"=w614:u32, "Left"=w613:i32, "Top"=w609:i32)  [unwired: 2 in, 2 out]
            n308 = Subtract(x=w609, y=5) -> (x-y=w607:i32)
            n309 = Compound Arithmetic op=ADD(w614, w613, 20 ("value")) -> (w621:u32)
            n310 = property on="Plot Selector" class="Ring (strict)"("Left"=w621, "Top"=w607) -> ()  [unwired: 2 in, 2 out]
          }
          frame 2 {
            n311 = property on="Current Godograph" class="XYGraph (strict)"() -> ("Position"=w653:T2)  [unwired: 2 in, 2 out]
            n312 = Unbundle By Name(w653) -> ("Left"=w652:i32, "Top"=w651:i32)
            n313 = Subtract(x=w652, y=20) -> (x-y=w630:i32)
            n314 = Subtract(x=w651, y=76) -> (x-y=w629:i32)
            n315 = Bundle By Name(cluster=w653, "Left"=w630, "Top"=w629) -> (w654:T2)
            n316 = Add(x=w630, y=20 ("Position:Left")) -> (x+y=w632:i32)
            n317 = Add(x=w629, y=10 ("Position:Top")) -> (x+y=w631:i32)
            n318 = property on="Pane" class="Pane"("Origin"=w654) -> ()  [unwired: 2 in, 2 out]
            n319 = property on="Choose file" class="Bool (strict)"("Left"=w632, "Top"=w631, "Height"=u32 65 ("Button Size:Height"), "Width"=u32 90 ("Button Size:Width")) -> ("Width"=w645:u32, "Left"=w644:i32, "Top"=w640:i32)  [unwired: 2 in, 2 out]
            n320 = Add(x=w640, y=25) -> (x+y=w638:i32)
            n321 = Compound Arithmetic op=ADD(w645, w644, 20 ("value")) -> (w643:u32)
            n322 = property on="Hold" class="Bool (strict)"("Left"=w643, "Top"=w638) -> ("Width"=w642:u32, "Left"=w641:i32, "Top"=w637:i32)  [unwired: 2 in, 2 out]
            n323 = Subtract(x=w637, y=5) -> (x-y=w635:i32)
            n324 = Compound Arithmetic op=ADD(w642, w641, 20 ("value")) -> (w649:u32)
            n325 = property on="Plot Selector" class="Ring (strict)"("Left"=w649, "Top"=w635) -> ()  [unwired: 2 in, 2 out]
          }
          frame 3 {
            n326 = property on="Voltage Godograph" class="XYGraph (strict)"() -> ("Position"=w683:T2)  [unwired: 2 in, 2 out]
            n327 = Unbundle By Name(w683) -> ("Left"=w682:i32, "Top"=w681:i32)
            n328 = Subtract(x=w682, y=20) -> (x-y=w658:i32)
            n329 = Subtract(x=w681, y=76) -> (x-y=w657:i32)
            n330 = Bundle By Name(cluster=w683, "Left"=w658, "Top"=w657) -> (w684:T2)
            n331 = Add(x=w658, y=20 ("Position:Left")) -> (x+y=w660:i32)
            n332 = Add(x=w657, y=10 ("Position:Top")) -> (x+y=w659:i32)
            n333 = property on="Pane" class="Pane"("Origin"=w684) -> ()  [unwired: 2 in, 2 out]
            n334 = property on="Choose file" class="Bool (strict)"("Left"=w660, "Top"=w659, "Height"=u32 65 ("Button Size:Height"), "Width"=u32 90 ("Button Size:Width")) -> ("Width"=w673:u32, "Left"=w672:i32, "Top"=w668:i32)  [unwired: 2 in, 2 out]
            n335 = Add(x=w668, y=25) -> (x+y=w666:i32)
            n336 = Compound Arithmetic op=ADD(w673, w672, 20 ("value")) -> (w671:u32)
            n337 = property on="Hold" class="Bool (strict)"("Left"=w671, "Top"=w666) -> ("Width"=w670:u32, "Left"=w669:i32, "Top"=w665:i32)  [unwired: 2 in, 2 out]
            n338 = Subtract(x=w665, y=5) -> (x-y=w663:i32)
            n339 = Compound Arithmetic op=ADD(w670, w669, 20 ("value")) -> (w677:u32)
            n340 = property on="Plot Selector" class="Ring (strict)"("Left"=w677, "Top"=w663) -> ()  [unwired: 2 in, 2 out]
          }
          frame 4 {
            n341 = property on="Current Spectrum" class="WFGraph (strict)"() -> ("Position"=w709:T2)  [unwired: 2 in, 2 out]
            n342 = Unbundle By Name(w709) -> ("Left"=w708:i32, "Top"=w707:i32)
            n343 = Subtract(x=w708, y=20) -> (x-y=w686:i32)
            n344 = Subtract(x=w707, y=76) -> (x-y=w685:i32)
            n345 = Bundle By Name(cluster=w709, "Left"=w686, "Top"=w685) -> (w710:T2)
            n346 = Add(x=w686, y=20 ("Position:Left")) -> (x+y=w688:i32)
            n347 = Add(x=w685, y=10 ("Position:Top")) -> (x+y=w687:i32)
            n348 = property on="Pane" class="Pane"("Origin"=w710) -> ()  [unwired: 2 in, 2 out]
            n349 = property on="Choose file" class="Bool (strict)"("Left"=w688, "Top"=w687, "Height"=u32 65 ("Button Size:Height"), "Width"=u32 90 ("Button Size:Width")) -> ("Width"=w701:u32, "Left"=w700:i32, "Top"=w696:i32)  [unwired: 2 in, 2 out]
            n350 = Add(x=w696, y=25) -> (x+y=w694:i32)
            n351 = Compound Arithmetic op=ADD(w701, w700, 20 ("value")) -> (w699:u32)
            n352 = property on="Hold" class="Bool (strict)"("Left"=w699, "Top"=w694) -> ("Width"=w698:u32, "Left"=w697:i32, "Top"=w693:i32)  [unwired: 2 in, 2 out]
            n353 = Subtract(x=w693, y=5) -> (x-y=w691:i32)
            n354 = Compound Arithmetic op=ADD(w698, w697, 20 ("value")) -> (w705:u32)
            n355 = property on="Plot Selector" class="Ring (strict)"("Left"=w705, "Top"=w691) -> ()  [unwired: 2 in, 2 out]
          }
          frame 5 {
            n356 = property on="Voltage Spectrum" class="WFGraph (strict)"() -> ("Position"=w737:T2)  [unwired: 2 in, 2 out]
            n357 = Unbundle By Name(w737) -> ("Left"=w736:i32, "Top"=w735:i32)
            n358 = Subtract(x=w736, y=20) -> (x-y=w714:i32)
            n359 = Subtract(x=w735, y=76) -> (x-y=w713:i32)
            n360 = Bundle By Name(cluster=w737, "Left"=w714, "Top"=w713) -> (w738:T2)
            n361 = Add(x=w714, y=20 ("Position:Left")) -> (x+y=w716:i32)
            n362 = Add(x=w713, y=10 ("Position:Top")) -> (x+y=w715:i32)
            n363 = property on="Pane" class="Pane"("Origin"=w738) -> ()  [unwired: 2 in, 2 out]
            n364 = property on="Choose file" class="Bool (strict)"("Left"=w716, "Top"=w715, "Height"=u32 65 ("Button Size:Height"), "Width"=u32 90 ("Button Size:Width")) -> ("Width"=w729:u32, "Left"=w728:i32, "Top"=w724:i32)  [unwired: 2 in, 2 out]
            n365 = Add(x=w724, y=25) -> (x+y=w722:i32)
            n366 = Compound Arithmetic op=ADD(w729, w728, 20 ("value")) -> (w727:u32)
            n367 = property on="Hold" class="Bool (strict)"("Left"=w727, "Top"=w722) -> ("Width"=w726:u32, "Left"=w725:i32, "Top"=w721:i32)  [unwired: 2 in, 2 out]
            n368 = Subtract(x=w721, y=5) -> (x-y=w719:i32)
            n369 = Compound Arithmetic op=ADD(w726, w725, 20 ("value")) -> (w733:u32)
            n370 = property on="Plot Selector" class="Ring (strict)"("Left"=w733, "Top"=w719) -> ()  [unwired: 2 in, 2 out]
          }
          frame 6 {
            n371 = property on="Current Park Spectrum" class="WFGraph (strict)"() -> ("Position"=w765:T2)  [unwired: 2 in, 2 out]
            n372 = Unbundle By Name(w765) -> ("Left"=w764:i32, "Top"=w763:i32)
            n373 = Subtract(x=w764, y=20) -> (x-y=w742:i32)
            n374 = Subtract(x=w763, y=76) -> (x-y=w741:i32)
            n375 = Bundle By Name(cluster=w765, "Left"=w742, "Top"=w741) -> (w766:T2)
            n376 = Add(x=w742, y=20 ("Position:Left")) -> (x+y=w744:i32)
            n377 = Add(x=w741, y=10 ("Position:Top")) -> (x+y=w743:i32)
            n378 = property on="Pane" class="Pane"("Origin"=w766) -> ()  [unwired: 2 in, 2 out]
            n379 = property on="Choose file" class="Bool (strict)"("Left"=w744, "Top"=w743, "Height"=u32 65 ("Button Size:Height"), "Width"=u32 90 ("Button Size:Width")) -> ("Width"=w757:u32, "Left"=w756:i32, "Top"=w752:i32)  [unwired: 2 in, 2 out]
            n380 = Add(x=w752, y=25) -> (x+y=w750:i32)
            n381 = Compound Arithmetic op=ADD(w757, w756, 20 ("value")) -> (w755:u32)
            n382 = property on="Hold" class="Bool (strict)"("Left"=w755, "Top"=w750) -> ("Width"=w754:u32, "Left"=w753:i32, "Top"=w749:i32)  [unwired: 2 in, 2 out]
            n383 = Subtract(x=w749, y=5) -> (x-y=w747:i32)
            n384 = Compound Arithmetic op=ADD(w754, w753, 20 ("value")) -> (w761:u32)
            n385 = property on="Plot Selector" class="Ring (strict)"("Left"=w761, "Top"=w747) -> ()  [unwired: 2 in, 2 out]
          }
          frame 7 {
            n386 = property on="Voltage Park Spectrum" class="WFGraph (strict)"() -> ("Position"=w793:T2)  [unwired: 2 in, 2 out]
            n387 = Unbundle By Name(w793) -> ("Left"=w792:i32, "Top"=w791:i32)
            n388 = Subtract(x=w792, y=20) -> (x-y=w772:i32)
            n389 = Subtract(x=w791, y=76) -> (x-y=w771:i32)
            n390 = Bundle By Name(cluster=w793, "Left"=w772, "Top"=w771) -> (w794:T2)
            n391 = Add(x=w772, y=20 ("Position:Left")) -> (x+y=w770:i32)
            n392 = Add(x=w771, y=10 ("Position:Top")) -> (x+y=w769:i32)
            n393 = property on="Pane" class="Pane"("Origin"=w794) -> ()  [unwired: 2 in, 2 out]
            n394 = property on="Choose file" class="Bool (strict)"("Left"=w770, "Top"=w769, "Height"=u32 65 ("Button Size:Height"), "Width"=u32 90 ("Button Size:Width")) -> ("Width"=w785:u32, "Left"=w784:i32, "Top"=w780:i32)  [unwired: 2 in, 2 out]
            n395 = Add(x=w780, y=25) -> (x+y=w778:i32)
            n396 = Compound Arithmetic op=ADD(w785, w784, 20 ("value")) -> (w783:u32)
            n397 = property on="Hold" class="Bool (strict)"("Left"=w783, "Top"=w778) -> ("Width"=w782:u32, "Left"=w781:i32, "Top"=w777:i32)  [unwired: 2 in, 2 out]
            n398 = Subtract(x=w777, y=5) -> (x-y=w775:i32)
            n399 = Compound Arithmetic op=ADD(w782, w781, 20 ("value")) -> (w789:u32)
            n400 = property on="Plot Selector" class="Ring (strict)"("Left"=w789, "Top"=w775) -> ()  [unwired: 2 in, 2 out]
          }
        }
      }
    }
  }
